vi "数字量输入.vi"(8 "CAN端口":u16, 10 "输入值":i16) -> ()   [LabVIEW 2010]
uses:
  全局量/试验配置信息.vi
panel:
  out "结束？":bool
  in  "同步_2":i32
  out "数据组数":i32
  in  "同步_1":i32
  # "0或1"
  # "从1 开始"
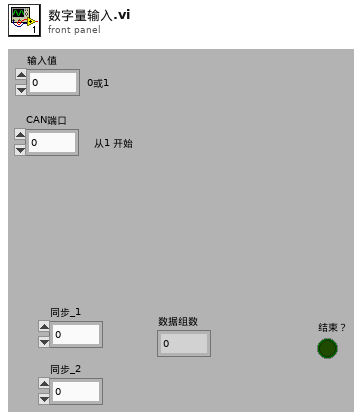
[diagram p1: front panel]
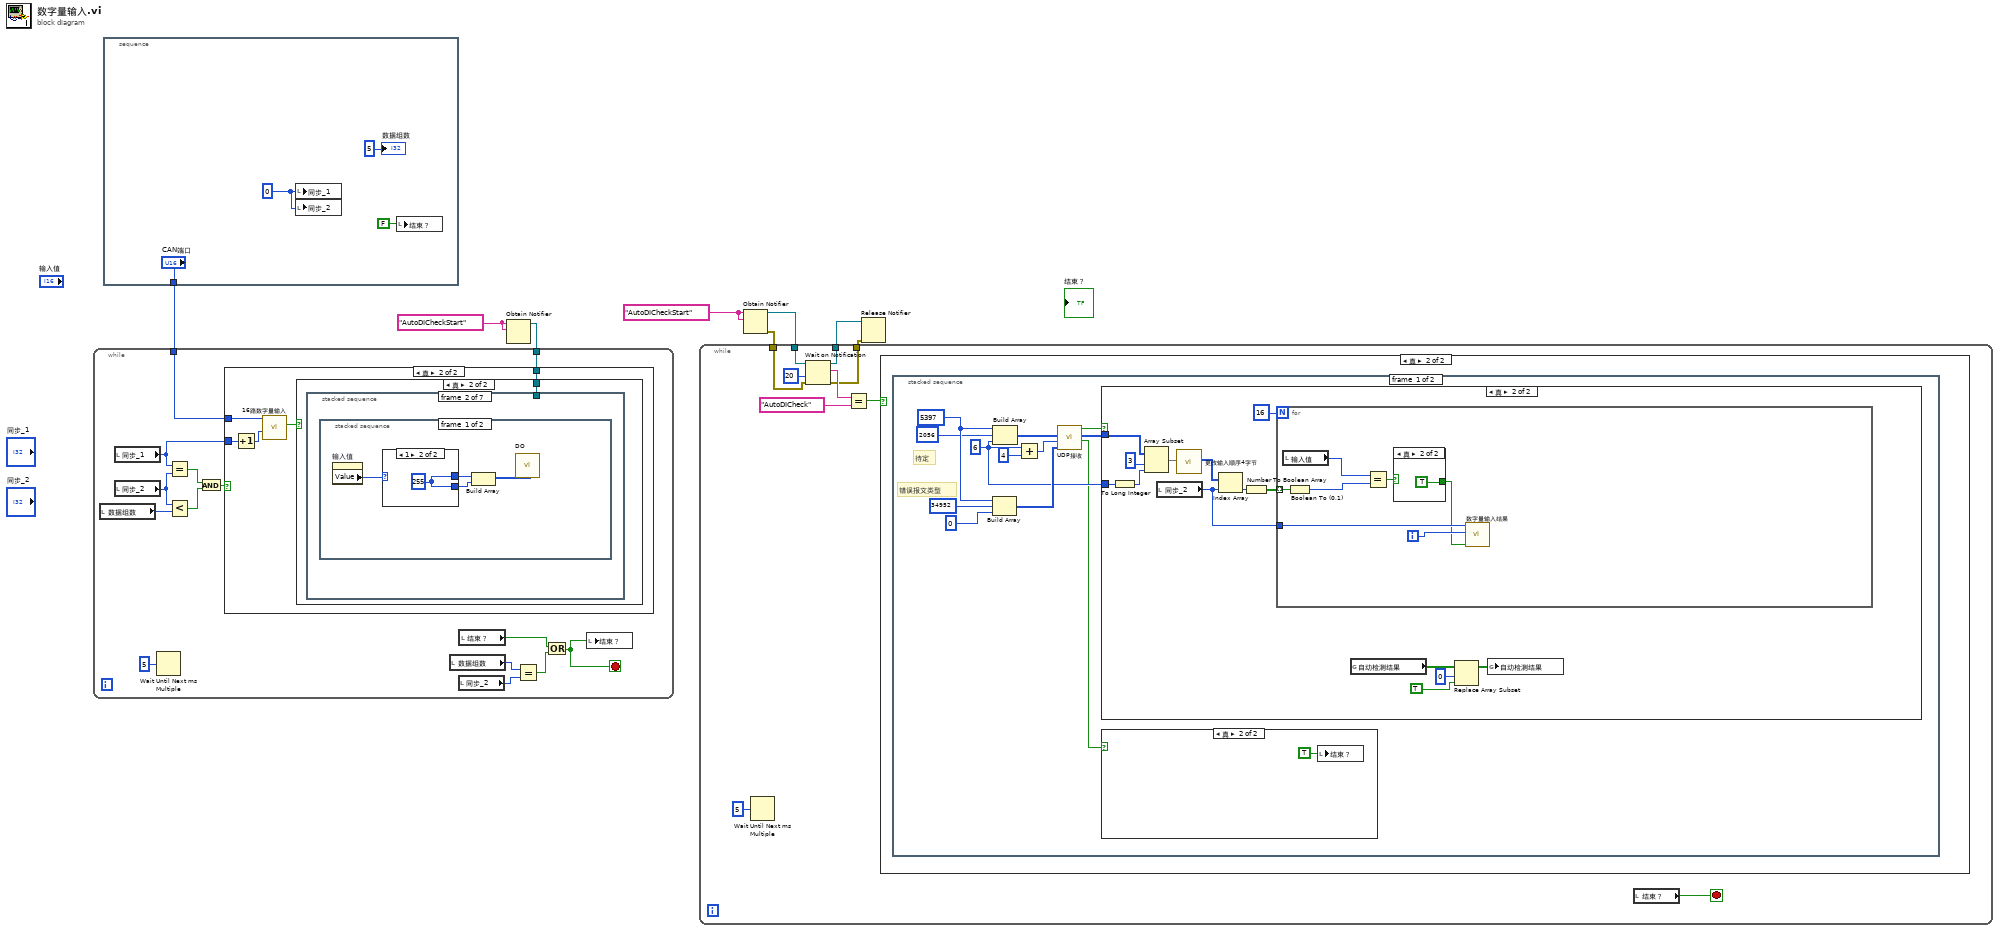
[diagram p0: block diagram]
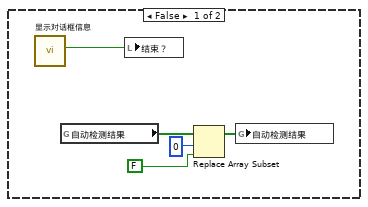
[diagram p3: hidden frame]
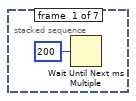
[diagram p4: hidden frame]
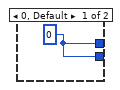
[diagram p5: hidden frame]
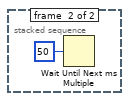
[diagram p6: hidden frame]
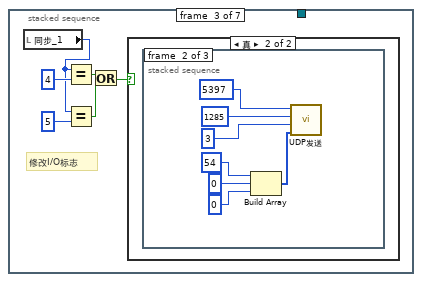
[diagram p7: hidden frame]
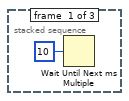
[diagram p9: hidden frame]
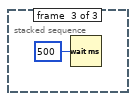
[diagram p10: hidden frame]
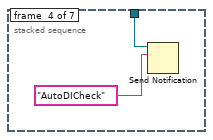
[diagram p11: hidden frame]
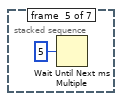
[diagram p12: hidden frame]
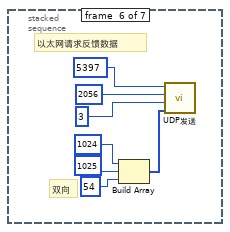
[diagram p13: hidden frame]
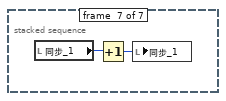
[diagram p14: hidden frame]
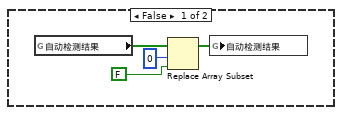
[diagram p17: hidden frame]
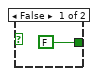
[diagram p18: hidden frame]
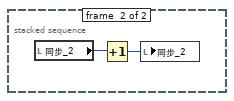
[diagram p19: hidden frame]
diagram:
  w3 = "AutoDICheckStart" ("名称（未命名）")
  w8 = "AutoDICheckStart" ("名称（未命名）")
  n1 = stacked-sequence {
    tunnel: ["CAN端口"] -> w1
    frame #0 {
      w12 = 0 ("同步_1")
      n2 = local write "同步_1"(w12) -> ()
      n3 = local write "同步_2"(w12) -> ()
      n4 = local write "结束？"(FALSE ("结束？")) -> ()
      "数据组数" <- 5 ("数据组数")
    }
  }
  n5 = Obtain Notifier(name (unnamed)=w3, notification data type=w3) -> (notifier out=w2:refnum<notifier>)  [unwired: 2 in, 2 out]
  n6 = while {
    tunnel: w2 -> [w14]
    tunnel: w1 -> [w13]
    stop <- w23 stop-if-true
    n7 = local read "数据组数"() -> (w18:i32)
    n8 = local read "同步_1"() -> (w20:i32)
    n9 = local read "同步_2"() -> (w19:i32)
    n10 = Wait Until Next ms Multiple(millisecond multiple=u32 5 ("毫秒倍数")) -> ()  [unwired: 1 out]
    n11 = Equal?(x=w20, y=w19) -> (x = y?=w16:bool)
    n12 = Less?(x=w19, y=w18) -> (x < y?=w15:bool)
    n13 = And(x=w16, y=w15) -> (x .and. y?=w17:bool)
    n14 = case shown="真" w17 {
      tunnel: w20 -> [_ w29]
      tunnel: w13 -> [_ w28]
      tunnel: w14 -> [_ w27]
      frame False {
      }
      frame True {
        n15 = Increment(x=w29) -> (x+1=w30:i32)
        n16 = call "16路数字量输入.vi"("第几组数据"=w30, "CAN端口"=w28) -> ("成功?"=w31:bool)  [unwired: 9 in]
        n17 = case shown="真" w31 {
          tunnel: w27 -> [_ w37]
          frame False {
            n18 = call "显示对话框信息"() -> ("确定"=w36:bool)  [unwired: 10 in, 1 out]
            n19 = global read "试验配置信息.vi" "自动检测结果"() -> (w33:bool[])
            n20 = local write "结束？"(w36) -> ()
            n21 = Replace Array Subset(array=w33, new element=FALSE, index=0 ("索引")) -> (w34:bool[])
            n22 = global write "试验配置信息.vi" "自动检测结果"(w34) -> ()
          }
          frame True {
            n23 = stacked-sequence {
              tunnel: w37 -> [_ _ _ w61 _ _ _]
              frame #0 {
                n24 = Wait Until Next ms Multiple(millisecond multiple=u32 200 ("毫秒倍数")) -> ()  [unwired: 1 out]
              }
              frame #1 {
                n25 = stacked-sequence {
                  frame #0 {
                    n26 = property on="输入值" class="DigNum (严格)"() -> ("Value"=w39:i16)  [unwired: 2 in, 2 out]
                    n27 = case shown="1" w39 {
                      tunnel: [w43 w44] -> w41
                      tunnel: [w43 w44] -> w40
                      frame 0, Default {
                        w43 = u8 0
                      }
                      frame 1 {
                        w44 = u8 255
                      }
                    }
                    n28 = Build Array(w41, w40) -> (w42:u8[])
                    n29 = call "DO"("dataIn(U8Array)"=w42) -> ()  [unwired: 2 in, 17 out]
                  }
                  frame #1 {
                    n30 = Wait Until Next ms Multiple(millisecond multiple=u32 50 ("毫秒倍数")) -> ()  [unwired: 1 out]
                  }
                }
              }
              frame #2 {
                # "修改I/O标志"
                n31 = local read "同步_1"() -> (w47:i32)
                n32 = Equal?(x=w47, y=4) -> (x = y?=w50:bool)
                n33 = Equal?(x=w47, y=5) -> (x = y?=w51:bool)
                n34 = Or(x=w50, y=w51) -> (x .or. y?=w46:bool)
                n35 = case shown="真" w46 {
                  frame False {
                  }
                  frame True {
                    n36 = stacked-sequence {
                      frame #0 {
                        n37 = Wait Until Next ms Multiple(millisecond multiple=u32 10 ("毫秒倍数")) -> ()  [unwired: 1 out]
                      }
                      frame #1 {
                        n38 = Build Array(u16 54, u16 0, u16 0) -> (w59:u16[])
                        n39 = call "UDP发送.vi"("发送数据"=w59, "数据区字长"=u16 3, "报文类型"=u16 1285, "发送方标识"=u16 5397) -> ()  [unwired: 6 in, 1 out]
                      }
                      frame #2 {
                        n40 = Wait (ms)(milliseconds to wait=u32 500 ("毫秒倍数")) -> ()  [unwired: 1 out]
                      }
                    }
                  }
                }
              }
              frame #3 {
                n41 = Send Notification(notification="AutoDICheck" ("通知"), notifier=w61) -> ()  [unwired: 1 in, 2 out]
              }
              frame #4 {
                n42 = Wait Until Next ms Multiple(millisecond multiple=u32 5 ("等待时间（毫秒）")) -> ()  [unwired: 1 out]
              }
              frame #5 {
                # "双向"
                # "以太网请求反馈数据"
                n43 = Build Array(u16 1024, u16 1025, u16 54) -> (w65:u16[])
                n44 = call "UDP发送.vi"("发送数据"=w65, "数据区字长"=u16 3, "报文类型"=u16 2056, "发送方标识"=u16 5397) -> ()  [unwired: 6 in, 1 out]
              }
              frame #6 {
                n45 = local read "同步_1"() -> (w72:i32)
                n46 = Increment(x=w72) -> (x+1=w71:i32)
                n47 = local write "同步_1"(w71) -> ()
              }
            }
          }
        }
      }
    }
    n48 = local read "数据组数"() -> (w24:i32)
    n49 = local read "同步_2"() -> (w25:i32)
    n50 = local read "结束？"() -> (w22:bool)
    n51 = Equal?(x=w24, y=w25) -> (x = y?=w21:bool)
    n52 = Or(x=w22, y=w21) -> (x .or. y?=w23:bool)
    n53 = local write "结束？"(w23) -> ()
  }
  n54 = Obtain Notifier(name (unnamed)=w8, notification data type=w8) -> (notifier out=w7:refnum<notifier>, error out=w5:errorcluster)  [unwired: 2 in, 1 out]
  n55 = while {
    tunnel: w7 -> [w79]
    tunnel: [w78] -> w6
    tunnel: w5 -> [w77]
    tunnel: [w76] -> w4
    stop <- w74 stop-if-true
    n56 = Wait Until Next ms Multiple(millisecond multiple=u32 5 ("毫秒倍数")) -> ()  [unwired: 1 out]
    n57 = Wait on Notification(notifier=w79, timeout in ms (-1)=20 ("超时毫秒(-1)"), error in (no error)=w77) -> (notifier out=w78:refnum<notifier>, notification=w82:string, error out=w76:errorcluster)  [unwired: 1 in, 1 out]
    n58 = Equal?(x=w82, y="AutoDICheck" ("通知")) -> (x = y?=w75:bool)
    n59 = case shown="真" w75 {
      frame False {
      }
      frame True {
        n60 = stacked-sequence {
          frame #0 {
            w84 = u16 6
            w89 = u16 5397
            # "错误报文类型"
            # "待定"
            n61 = Build Array(w89, u16 34952, u16 0 ("元素")) -> (w92:u16[])
            n62 = Build Array(w89, u16 2056, w84) -> (w88:u16[])
            n63 = Add(x=w84, y=u16 4) -> (x+y=w94:u16)
            n64 = call "UDP接收.vi"("匹配帧信息_异常"=w92, "长度"=w94, "匹配帧信息_正常"=w88) -> ("接收超时?"=w83:bool, "接收的一帧数据"=w85:u16[], "正常_找到?"=w86:bool)  [unwired: 5 in, 1 out]
            n65 = case shown="真" w86 {
              tunnel: w85 -> [_ w111]
              tunnel: w84 -> [_ w110]
              frame False {
                n66 = global read "试验配置信息.vi" "自动检测结果"() -> (w98:bool[])
                n67 = Replace Array Subset(array=w98, new element=FALSE, index=0 ("索引")) -> (w97:bool[])
                n68 = global write "试验配置信息.vi" "自动检测结果"(w97) -> ()
              }
              frame True {
                n69 = To Long Integer(number=w110) -> (32bit integer=w113:i32)
                n70 = Array Subset(array=w111, index=3 ("索引"), length=w113) -> (w109:u16[])
                n71 = local read "同步_2"() -> (w104:i32)
                n72 = call "更改输入顺序4字节.vi"("输入数据"=w109) -> ("更改顺序后数据"=w108:u16[])  [unwired: 10 in]
                n73 = Index Array(array=w108, index=w104) -> (element=w107:u16)
                n74 = Number To Boolean Array(number=w107) -> (Boolean array=w106:bool[])
                n75 = for {
                  N: 16 -> [_]
                  tunnel: w106 -> [w120] mode=indexing
                  tunnel: w104 -> [w116]
                  i -> [w115]
                  n76 = local read "输入值"() -> (w118:i16)
                  n77 = Boolean To (0,1)(Boolean=w120) -> (0, 1=w117:i16)
                  n78 = Equal?(x=w118, y=w117) -> (x = y?=w119:bool)
                  n79 = case shown="真" w119 {
                    tunnel: [FALSE TRUE] -> w114
                    frame False {
                    }
                    frame True {
                    }
                  }
                  n80 = call "数字量输入结果.vi"("合格?"=w114, "第几个"=w115, "第几组"=w116) -> ()  [unwired: 9 in]
                }
                n81 = global read "试验配置信息.vi" "自动检测结果"() -> (w102:bool[])
                n82 = Replace Array Subset(array=w102, new element=TRUE, index=0 ("索引")) -> (w101:bool[])
                n83 = global write "试验配置信息.vi" "自动检测结果"(w101) -> ()
              }
            }
            n84 = case shown="真" w83 {
              frame False {
              }
              frame True {
                n85 = local write "结束？"(TRUE ("结束？")) -> ()
              }
            }
          }
          frame #1 {
            n86 = local read "同步_2"() -> (w124:i32)
            n87 = Increment(x=w124) -> (x+1=w123:i32)
            n88 = local write "同步_2"(w123) -> ()
          }
        }
      }
    }
    n89 = local read "结束？"() -> (w74:bool)
  }
  n90 = Release Notifier(notifier=w6, error in (no error)=w4) -> ()  [unwired: 1 in, 3 out]
